vi "Untitled 1.vi"() -> ()   [LabVIEW 2018]
panel:
  in  "Boolean":bool
  in  "Numeric":dbl
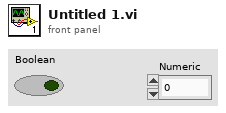
[diagram p1: front panel]
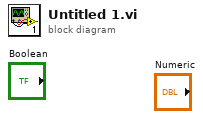
[diagram p0: block diagram]
diagram:
